vi "Acquire Sample Sets.vi"(8 "error in (no error)":errorcluster) -> (0 "error out":errorcluster, 2 "Sample Set":dbl[][](array[numeric]))   [LabVIEW 2011]
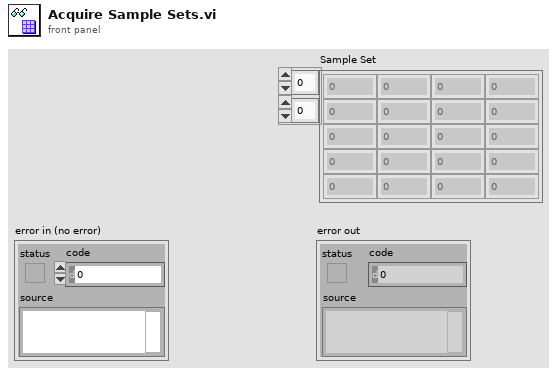
[diagram p1: front panel]
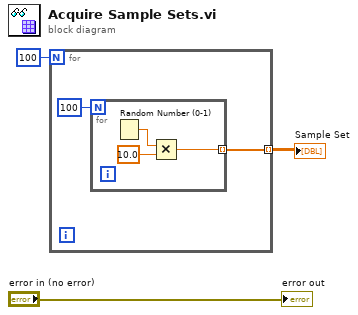
[diagram p0: block diagram]
diagram:
  n1 = for {
    N: 100 -> [_]
    tunnel: [w4] -> w2 mode=indexing
    n2 = for {
      N: 100 -> [_]
      tunnel: [w6] -> w4 mode=indexing
      n3 = Random Number (0-1)() -> (number: 0 to 1=w8:dbl)
      n4 = Multiply(x=w8, y=10.0) -> (x*y=w6:dbl)
    }
  }
  "Sample Set" <- w2
  "error out" <- "error in (no error)"
